vi "Hybrid Start Read Server.vi"() -> (0 "error out":errorcluster, 1 "dup reference":refnum<vi>)   [LabVIEW 2021]
doc: "This is a simple example of a server which exports VIs to be called from another machine. You may run both the client.llb and server.llb on the same machine without modifying the access list. If you wish to run the client on another machine that is not in your domain you will have to list the name of the client in the Machine Access List. \n\nThe VIs listed in the Exported VI list are exported by the server.\n\nTo run this example start this VI First, then start the client.llb on all machines you want to try as clients. If you change either of the above lists, you must restart this VI for the changes to take effect.\n\nClick the \"Stop\" button to quit. This will turn off the server, terminating all client connections, and restore the previous access lists to their original values."
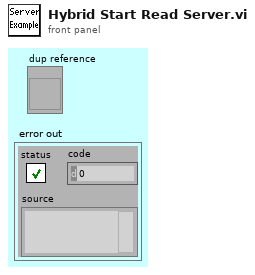
[diagram p1: front panel]
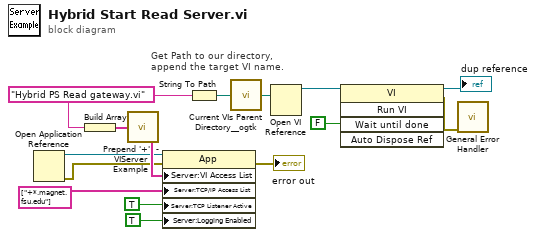
[diagram p0: block diagram]
diagram:
  w3 = "Hybrid PS Read gateway.vi"
  # "Get Path to our directory,\nappend the target VI name."
  n1 = Open Application Reference() -> (0:w7:errorcluster, 3:w8:refnum<vi>)  [unwired: 4 in]
  n2 = Build Array(w3) -> (w12:string[])
  n3 = call "Prepend '+'  - VIServer Example.vi"("list in"=w12) -> ("list out"=w15:string[])
  n4 = property class="App"(reference=w8, error in=w7, "Server:VI Access List"=w15, "Server:TCP/IP Access List"=string[] ["+*.magnet.fsu.edu"], "Server:TCP Listener Active"=TRUE ("Srvr.TCPActive"), "Server:Logging Enabled"=TRUE ("Srvr.LogEnabled")) -> (error out=→"error out":errorcluster)  [unwired: 1 out]
  n5 = String To Path(string=w3) -> (path=w2:path)
  n6 = call <userlib>:"Current VIs Parent Directory__ogtk.vi"("Relative path (.)"=w2) -> ("Parent Directory (+ Relative)"=w1:path)  [unwired: 4 in]
  n7 = Open VI Reference(vi path=w1) -> (vi reference=w5:refnum<vi>)  [unwired: 5 in, 1 out]
  n8 = invoke class="VI" method="Run VI"(reference=w5, "Wait until done"=FALSE) -> (reference out=→"dup reference":refnum<vi>, error out=w10:errorcluster)  [unwired: 3 in, 3 out]
  n9 = call <vilib>:"General Error Handler.vi"("error in (no error)"=w10) -> ()  [unwired: 10 in, 5 out]
